vi "Install Octave Package golpi.vi"(6 "Verbose? (T)":bool=TRUE, 7 "Feature name":string="Bitstream data transfer mode", 8 "error in":errorcluster, 11 "GOLPI ref. in":T1={"pipe handle"={"lv_proc.dll file path"=path "", "process instance handle"=[], "debug mode"=FALSE, "debug data"=[]}, "fast read timeout [ms]"=500, "fast read settle time [ms]"=10, "fast read to multiple [ms]"=1, "max elements per input line"=100, "slow read timeout [ms]"=5000, "stdin double format specifier"="", "max elements per stdout output column"=100, "console mode bitstream"=FALSE, "bitstream first read timeout [ms]"=1000, "bitstream read timeout [ms]"=50, "struct transfer possible"=FALSE, "matlab mode"=FALSE}) -> (0 "error out":errorcluster, 3 "GOLPI ref. out":T1={"pipe handle"={"lv_proc.dll file path"=path "", "process instance handle"=[], "debug mode"=FALSE, "debug data"=[]}, "fast read timeout [ms]"=500, "fast read settle time [ms]"=10, "fast read to multiple [ms]"=1, "max elements per input line"=100, "slow read timeout [ms]"=5000, "stdin double format specifier"="", "max elements per stdout output column"=100, "console mode bitstream"=FALSE, "bitstream first read timeout [ms]"=1000, "bitstream read timeout [ms]"=50, "struct transfer possible"=FALSE, "matlab mode"=FALSE})   [LabVIEW 2020, in "GOLPI library.lvlib"]
doc: "Install GNU Octave package golpi. This package is required for Bitstream data transfer mode and for transfer of GNU Octave structures to LabVIEW clusters. VI search for package file golpi-X.X.X.tar.gz in application directory and subdirectories. If not found, a file dialog is opened for user to determine position of file. Input \"Feature name\" is used in description of message box. Input Verbose disables message box and file dialog.\n\n---\nGOLPI works only with lv_proc.dll library, which is part of vipm package or should be delivered together with packed library. Placement of this dll is selected in terminal of Start GNU Octave.vi."
uses:
  GOLPI library.lvlib
  GOLPI reference Type Def.ctl
  Pipe Handle.ctl
  Custom Error Codes Enum Type Def.vi
  <vilib>/regexp/Match Regular Expression.xnode
  LV Process library.lvlib
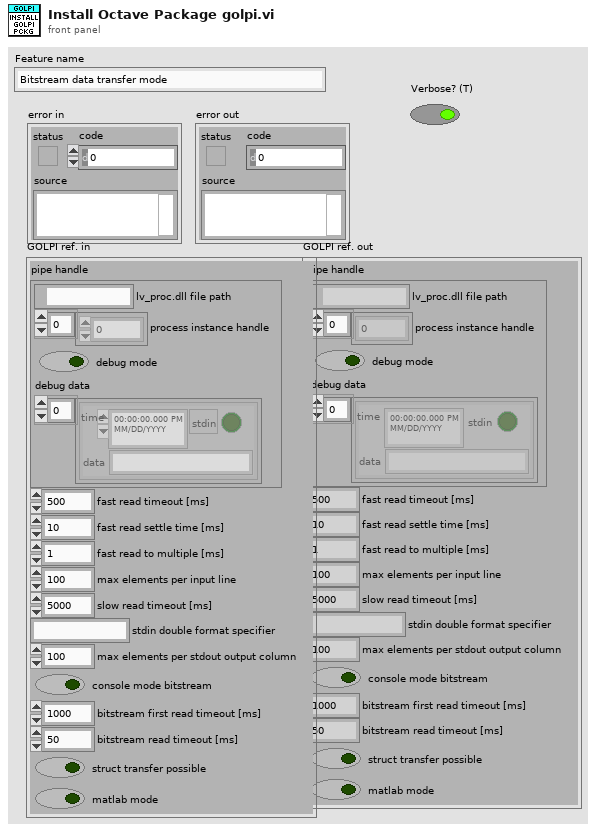
[diagram p1: front panel]
types:
  T1 = typedef "GOLPI library.lvlib/GOLPI reference Type Def.ctl" = cluster{"pipe handle":T2, "fast read timeout [ms]":u32, "fast read settle time [ms]":u32, "fast read to multiple [ms]":u32, "max elements per input line":u32, "slow read timeout [ms]":u32, "stdin double format specifier":string, "max elements per stdout output column":u32, "console mode bitstream":bool, "bitstream first read timeout [ms]":u32, "bitstream read timeout [ms]":u32, "struct transfer possible":bool, "matlab mode":bool}
  T2 = typedef "LV Process library.lvlib/Pipe Handle.ctl" = cluster{"lv_proc.dll file path":path, "process instance handle":u32[], "debug mode":bool, "debug data":cluster{"time":timestamp, "stdin":bool, "data":string}[]}
  T3 = typedef "GOLPI library.lvlib/Custom Error Codes Enum Type Def.vi" = enum16{"no error", "00 working directory PAR1 missing", "01 octave binary PAR1 missing", "02 octave report error PAR1", "03 empty output last cmd PAR1", "04 missing temporary file PAR1", "05 pwd PAR 1 not exist", "06 oct package not installed", "07 octave default binary missing", "10 var PAR1 not string, vect", "11 var PAR1 not num, scal, ~compl", "12 var PAR1 not num, scal, compl", "13 var PAR1 not num, vect, ~compl", "14 var PAR1 not num, vect, compl", "15 var PAR1 not num, mat, ~compl", "16 var PAR1 not num, mat, ~compl", "30 read timeout", "60 bitstream transport failed", "61 bitstream decode error PAR1", "62 bitstream cannot be set", "70 struct transfer not possible", "80 struct: cluster elem. PAR1 not implem.", "81 struct: structure field PAR1 not implem.", "82 struct: size mismatch of PAR1", "83 struct: type mismatch of PAR1", "98 internal error", "99 not finished", "90 Not supported in Matlab mode", "91 Matlab variable transfer error", "92 Matlab Script Error"}
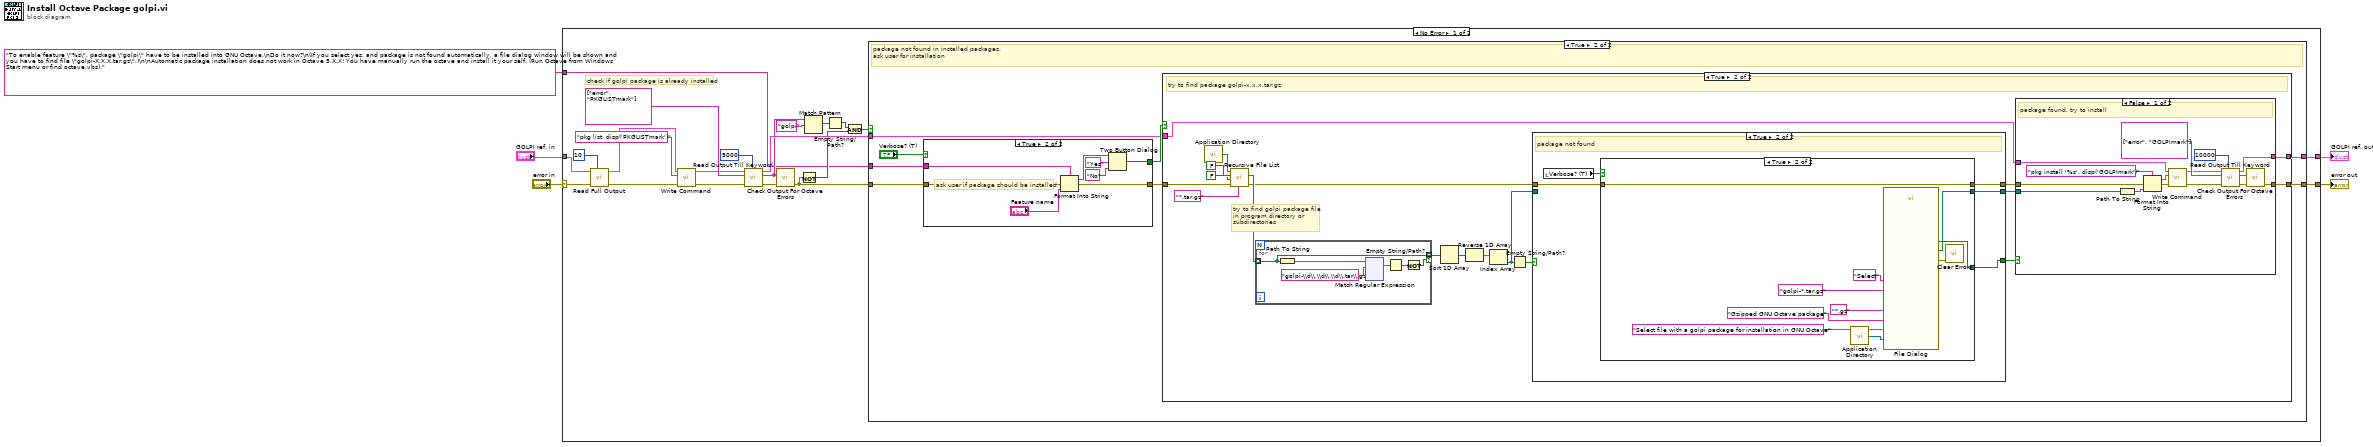
[diagram p0: block diagram]
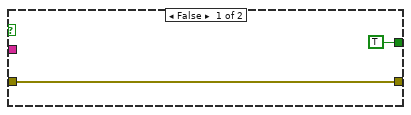
[diagram p3: hidden frame]
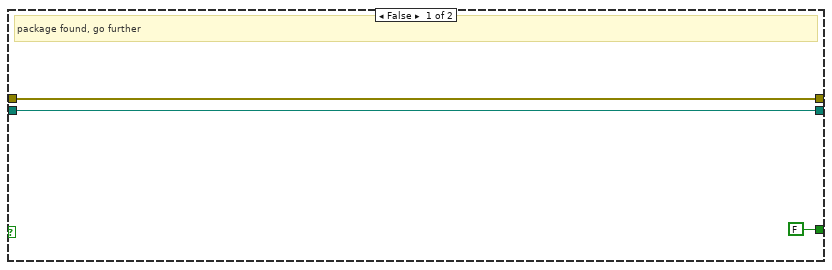
[diagram p5: hidden frame]
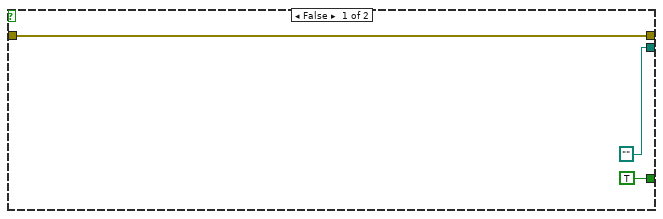
[diagram p6: hidden frame]
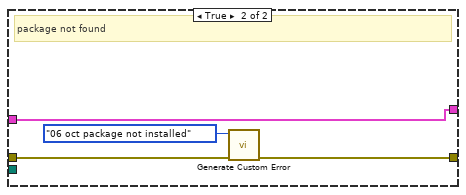
[diagram p7: hidden frame]
diagram:
  n1 = case shown="No Error" "error in" {
    selector: "error in" -> [w26 w229]
    tunnel: "GOLPI ref. in" -> [w27 w228]
    tunnel: [w13 w228] -> w4
    tunnel: [w25 w229] -> w2
    tunnel: "To enable feature \"%s\", package \"golpi\" have to be installed into GNU Octave.\nDo it now?\n(If you select yes, and package is not found automatically, a file dialog window will be shown and you have to find file \"golpi-X.X.X.tar.gz\".)\n\nAutomatic package installation does not work in Octave 5.X.X! You have manually run the octave and install it your self. (Run Octave from Windows Start menu or find octave.vbs)." ("message") -> [w6 _]
    frame No Error {
      # "check if golpi package is already installed"
      n2 = call "Read Full Output.vi"("timeout [ms]"=u32 10, "error in"=w26, "GOLPI ref. in"=w27) -> ("error out"=w23:errorcluster, "GOLPI ref. out"=w24:T1)  [unwired: 5 in, 2 out]
      n3 = call "Write Command.vi"("error in"=w23, "command"="pkg list, disp('PKGLISTmark')", "GOLPI ref. in"=w24) -> ("error out"=w19:errorcluster, "GOLPI ref. out"=w18:T1)  [unwired: 7 in]
      n4 = call "Read Output Till Keyword.vi"("timeout [ms]"=u32 5000, "error in"=w19, "keywords"=string[] ["error", "PKGLISTmark"], "GOLPI ref. in"=w18) -> ("error out"=w10:errorcluster, "read buffer"=w9:string, "GOLPI ref. out"=w14:T1)  [unwired: 4 in, 1 out]
      n5 = call "Check Output For Octave Errors.vi"("error in"=w10, "read buffer"=w9) -> ("error out"=w8:errorcluster)  [unwired: 9 in]
      n6 = Not(x=w8) -> (.not. x?=w7:bool)
      n7 = Match Pattern(string=w9, regular expression="golpi") -> (match substring=w11:string)  [unwired: 1 in, 3 out]
      n8 = Empty String/Path?(string/path=w11) -> (empty?=w20:bool)
      n9 = Compound Arithmetic op=AND(w20, w7) -> (w16:bool)
      n10 = case shown="True" w16 {
        tunnel: [w29 w33] -> w25
        tunnel: w8 -> [w29 w37]
        tunnel: w14 -> [w28 w34]
        tunnel: [w28 w32] -> w13
        tunnel: w6 -> [_ w30]
        frame False {
          # "package seems to be already installed,\nnothing to do"
        }
        frame True {
          # "package not found in installed packages,\nask user for installation"
          n11 = case shown="True" "Verbose? (T)" {
            tunnel: w37 -> [w38 w45]
            tunnel: [TRUE ("T button?") w42] -> w36
            tunnel: [w38 w41] -> w35
            tunnel: w30 -> [_ w40]
            frame False {
            }
            frame True {
              # "ask user if package should be installed"
              n12 = Format Into String(format string=w40, error in=w45, "Feature name") -> (resulting string=w43:string, error out=w41:errorcluster)  [unwired: 1 in]
              n13 = Two Button Dialog(message=w43, 1:"No" ("F button name (\"Cancel\")"), 2:"Yes" ("T button name (\"OK\")")) -> (T button?=w42:bool)
            }
          }
          n14 = case shown="True" w36 {
            tunnel: w35 -> [w49 w54]
            tunnel: w34 -> [w48 w62]
            tunnel: [w49 w51] -> w33
            tunnel: [w48 w50] -> w32
            frame False {
              # "user do not want to install package, nothing to do, no error to generate."
            }
            frame True {
              # "try to find golpi package file\nin program directory or\nsubdirectories"
              # "try to find package golpi-x.x.x.tar.gz"
              n15 = call <vilib>:"Application Directory.vi"() -> ("Application Directory"=w67:path)
              n16 = call <vilib>:"Recursive File List.vi"("pattern"="*.tar.gz", "error in (no error)"=w54, "Continue Recursing on Error? (F)"=FALSE, "Treat LLBs as Folders?"=FALSE, "Folder Path"=w67) -> ("error out"=w53:errorcluster, "All Files in Dir"=w66:path[])  [unwired: 2 in, 3 out]
              n17 = for {
                tunnel: w66 -> [w110] mode=indexing
                tunnel: [w110] -> w65 mode=indexing if=w109
                n18 = Path To String(path=w110) -> (string=w108:string)
                n19 = xnode "Match Regular Expression"("input string"=w108, "regular expression"="golpi-\\d\\.\\d\\.\\d\\.tar\\.gz") -> ("whole match"=w112:string)  [unwired: 4 in, 4 out]
                n20 = Empty String/Path?(string/path=w112) -> (empty?=w111:bool)
                n21 = Not(x=w111) -> (.not. x?=w109:bool)
              }
              n22 = Sort 1D Array(array=w65) -> (sorted array=w64:path[])
              n23 = Reverse 1D Array(array=w64) -> (reversed array=w63:path[])
              n24 = Index Array(array=w63) -> (element=w59:path)  [unwired: 1 in]
              n25 = Empty String/Path?(string/path=w59) -> (empty?=w61:bool)
              n26 = case shown="True" w61 {
                tunnel: [FALSE w75] -> w60
                tunnel: [w69 w74] -> w58
                tunnel: w59 -> [w69 _]
                tunnel: w53 -> [w68 w73]
                tunnel: [w68 w72] -> w57
                frame False {
                  # "package found, go further"
                }
                frame True {
                  # "package not found"
                  n27 = local read "Verbose? (T)"() -> (w71:bool)
                  n28 = case shown="True" w71 {
                    tunnel: [TRUE ("cancelled") w82] -> w75
                    tunnel: [path "" w81] -> w74
                    tunnel: w73 -> [w78 w80]
                    tunnel: [w78 w80] -> w72
                    frame False {
                    }
                    frame True {
                      n29 = call <vilib>:"Application Directory.vi"() -> ("Application Directory"=w83:path)
                      n30 = call "File Dialog"("start path"=w83, "prompt"="Select file with a golpi package for installation in GNU Octave", "button label"="Select", "default name"="golpi-*.tar.gz", "pattern (all files)"="*.gz", "pattern label"="Gzipped GNU Octave package") -> ("selected path"=w81:path, "cancelled"=w82:bool, "error out"=w79:errorcluster)  [unwired: 6 in, 1 out]
                      n31 = call <vilib>:"Clear Errors.vi"("error in (no error)"=w79) -> ()  [unwired: 5 in, 2 out]
                    }
                  }
                }
              }
              n32 = case shown="False" w60 {
                tunnel: w57 -> [w92 w105]
                tunnel: w62 -> [w97 w107]
                tunnel: w58 -> [w96 _]
                tunnel: [w90 w104] -> w51
                tunnel: [w89 w107] -> w50
                frame False {
                  # "package found, try to install"
                  n33 = Path To String(path=w96) -> (string=w94:string)
                  n34 = Format Into String(format string="pkg install '%s', disp('GOLPImark')" ("command"), error in=w92, w94) -> (resulting string=w93:string, error out=w91:errorcluster)  [unwired: 1 in]
                  n35 = call "Write Command.vi"("error in"=w91, "command"=w93, "GOLPI ref. in"=w97) -> ("error out"=w102:errorcluster, "GOLPI ref. out"=w101:T1)  [unwired: 7 in]
                  n36 = call "Read Output Till Keyword.vi"("timeout [ms]"=u32 10000, "error in"=w102, "keywords"=string[] ["error", "GOLPImark"], "GOLPI ref. in"=w101) -> ("error out"=w99:errorcluster, "read buffer"=w98:string, "GOLPI ref. out"=w89:T1)  [unwired: 4 in, 1 out]
                  n37 = call "Check Output For Octave Errors.vi"("error in"=w99, "read buffer"=w98) -> ("error out"=w90:errorcluster)  [unwired: 9 in]
                }
                frame True {
                  # "package not found"
                  n38 = call "Generate Custom Error.vi"("error in"=w105, "GOLPI error"=Custom_Error_Codes_Enum_Type_Def.vi."06 oct package not installed") -> ("error out"=w104:errorcluster)  [unwired: 9 in]
                }
              }
            }
          }
        }
      }
    }
    frame Error {
    }
  }
  "error out" <- w2
  "GOLPI ref. out" <- w4
